vi "save_PES_image.vi"(13 "Image Data In":T1) -> ()   [LabVIEW 2023]
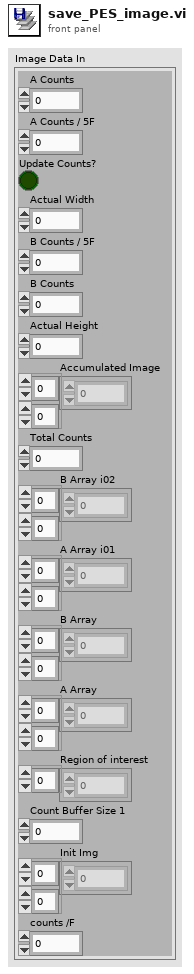
[diagram p1: front panel]
types:
  T1 = cluster{"A Counts":i32, "A Counts / 5F":dbl, "Update Counts?":bool, "Actual Width":u32, "B Counts / 5F ":dbl, "B Counts":i32, "Actual Height":u32, "Accumulated Image ":i16[][], "Total Counts":i32, "B Array i02":sgl[][], "A Array i01":sgl[][], "B Array":i16[][], "A Array":i16[][], "Region of interest":i32[], "Count Buffer Size 1":i32, "Init Img":i16[][], "counts /F":i16}
  T2 = enum16{"Left Button", "Center Button", "Right Button", "Window Close"}
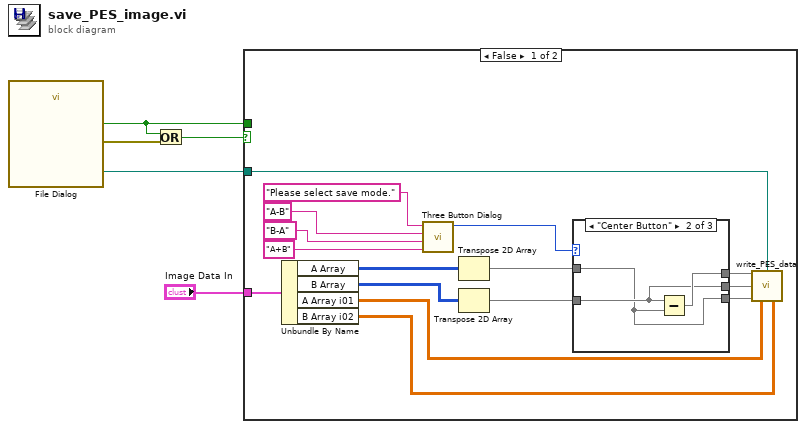
[diagram p0: block diagram]
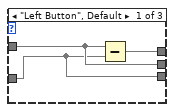
[diagram p2: hidden frame]
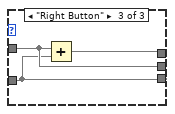
[diagram p3: hidden frame]
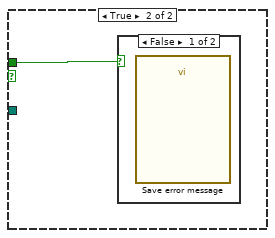
[diagram p4: hidden frame]
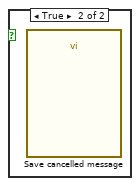
[diagram p5: hidden frame]
diagram:
  n1 = call "File Dialog"() -> ("selected path"=w5:path, "cancelled"=w2:bool, "error out"=w3:errorcluster)  [unwired: 12 in, 1 out]
  n2 = Or(x=w2, y=w3) -> (x .or. y?=w4:bool)
  n3 = case shown="False" w4 {
    tunnel: w5 -> [w11 _]
    tunnel: w2 -> [_ w31]
    tunnel: "Image Data In" -> [w10 _]
    frame False {
      n4 = Unbundle By Name(w10) -> ("A Array"=w9:i16[][], "B Array"=w8:i16[][], "A Array i01"=w7:sgl[][], "B Array i02"=w6:sgl[][])
      n5 = call <vilib>:"Three Button Dialog.vi"("Right Button Text (\"Cancel\")"="A+B" ("Right Button Text (\"Cancel\")"), "Center Button Text (\"No\")"="B-A" ("Center Button Text (\"No\")"), "Left Button Text (\"Yes\")"="A-B", "message"="Please select save mode.") -> ("Which Button?"=w19:T2)  [unwired: 7 in]
      n6 = Transpose 2D Array(2D array=w9) -> (transposed array=w20:i16[][])
      n7 = Transpose 2D Array(2D array=w8) -> (transposed array=w21:i16[][])
      n8 = case shown="\"Center Button\"" w19 {
        tunnel: w20 -> [w23 w25 w29]
        tunnel: w21 -> [w22 w26 w28]
        tunnel: [w24 w27 w30] -> w14
        tunnel: [w23 w26 w29] -> w13
        tunnel: [w22 w25 w28] -> w12
        frame "Left Button", Default {
          n9 = Subtract(x=w23, y=w22) -> (x-y=w24:i16[][])
        }
        frame "Center Button" {
          n10 = Subtract(x=w26, y=w25) -> (x-y=w27:i16[][])
        }
        frame "Right Button" {
          n11 = Add(x=w29, y=w28) -> (x+y=w30:i16[][])
        }
      }
      n12 = call "write_PES_data.vi"("Img-Bgd Data"=w14, "Path"=w11, "Img Data"=w13, "Bgd Data"=w12, "i01 Data"=w7, "i02 Data"=w6) -> ()  [unwired: 10 in]
    }
    frame True {
      n13 = case shown="False" w31 {
        frame False {
          n14 = call "Save error message"() -> ()  [unwired: 10 in, 2 out]
        }
        frame True {
          n15 = call "Save cancelled message"() -> ()  [unwired: 10 in, 2 out]
        }
      }
    }
  }
